vi "Wmeter Read.vi"(8 "error in":errorcluster, 11 "WMeter":refnum<visa-resource-name>) -> (0 "error out":errorcluster, 2 "Wavelength":dbl, 3 "WMeter out":refnum<visa-resource-name>)   [LabVIEW 2012]
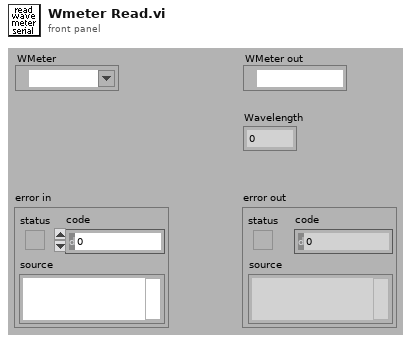
[diagram p1: front panel]
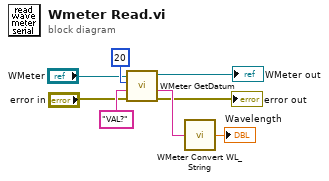
[diagram p0: block diagram]
diagram:
  n1 = call "WMeter GetDatum.vi"("error in"="error in", "Command"="VAL?" ("data"), "Wait W -> R (ms)"=u32 20 ("Delay Time (s)"), "WMeter"="WMeter") -> ("error out"=→"error out":errorcluster, "DataRead"=w6:string, "WMeter"=→"WMeter out":refnum<visa-resource-name>)  [unwired: 5 in]
  n2 = call "WMeter Convert WL_String.vi"("WL-String"=w6) -> ("Wavelength"=→"Wavelength":dbl)  [unwired: 4 in]
